vi "Write Future.vi"(8 "error in (no error)":errorcluster, 10 "Value":variant, 11 "Future in":refnum<class "Future.lvclass">) -> (0 "error out":errorcluster, 3 "Future out":refnum<class "Future.lvclass">)   [LabVIEW 2017, in "Promise Future.lvlib" / "Future.lvclass"]
uses:
  Future.lvclass
  Future.lvclass/Future.ctl
  c83e476c-f45e-459d-a1f3-ff7c88da77de.vi
  0608d02a-fc2f-4e6c-95dc-dd199133773d.vi
  Read Value.vi
  Value Set Callback.vi
  Wrapper VI Name.vi
  Then.vi
  <vilib>/Utility/error.llb/Error Cluster From Error Code.vi
  <vilib>/ErrorRing/Error Ring.xnode
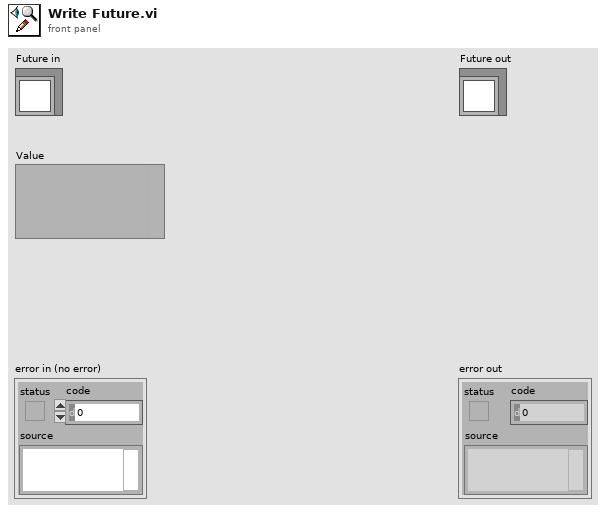
[diagram p1: front panel]
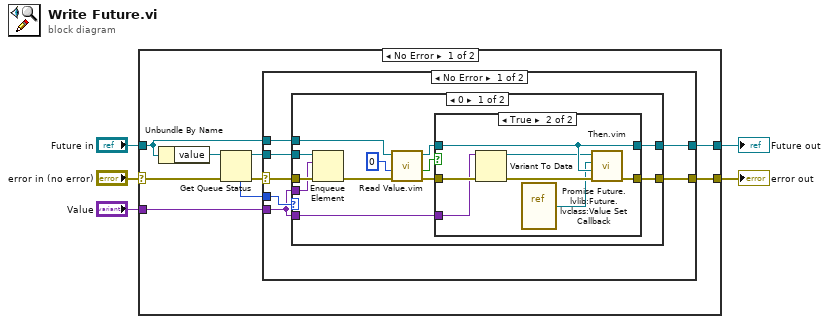
[diagram p0: block diagram]
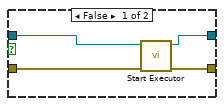
[diagram p2: hidden frame]
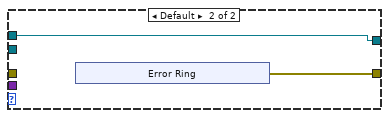
[diagram p3: hidden frame]
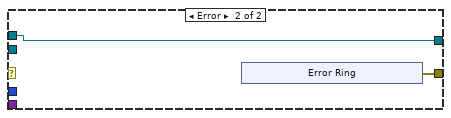
[diagram p4: hidden frame]
diagram:
  n1 = case shown="No Error" "error in (no error)" {
    selector: "error in (no error)" -> [w8 w60]
    tunnel: [w6 w60] -> w4
    tunnel: [w7 w59] -> w2
    tunnel: "Future in" -> [w10 w59]
    tunnel: "Value" -> [w9 _]
    frame No Error {
      n2 = Unbundle By Name(w10) -> ("value"=w11:refnum<queue>)
      n3 = Get Queue Status(queue=w11, error in (no error)=w8) -> (queue out=w13:refnum<queue>, error out=w14:errorcluster, # elements in queue=w12:i32)  [unwired: 1 in, 5 out]
      n4 = case shown="No Error" w14 {
        selector: w14 -> [w16 _]
        tunnel: [w21 w52] -> w6
        tunnel: w10 -> [w20 w53]
        tunnel: [w19 w53] -> w7
        tunnel: w12 -> [w18 _]
        tunnel: w13 -> [w17 _]
        tunnel: w9 -> [w15 _]
        frame No Error {
          n5 = case shown="0" w18 {
            tunnel: w20 -> [w28 w46]
            tunnel: w16 -> [w32 _]
            tunnel: [w29 w45] -> w21
            tunnel: [w30 w46] -> w19
            tunnel: w15 -> [w31 _]
            tunnel: w17 -> [w33 _]
            tunnel: w15 -> [w22 _]
            frame 0 {
              n6 = Enqueue Element(queue=w33, element=w31, error in (no error)=w32) -> (error out=w27:errorcluster)  [unwired: 1 in, 2 out]
              n7 = call "Read Value.vim"("error in (no error)"=w27, "timeout in ms (-1)"=0, "Future in"=w28) -> ("error out"=w26:errorcluster, "timed out?"=w24:bool, "Future out"=w25:refnum<class "Future.lvclass">)  [unwired: 5 in, 1 out]
              n8 = case shown="True" w24 {
                tunnel: [w37 w44] -> w30
                tunnel: [w36 w43] -> w29
                tunnel: w26 -> [w35 w41]
                tunnel: w25 -> [w34 w44]
                tunnel: w22 -> [_ w39]
                frame False {
                  n9 = call "Start Executor.vi"("error in (no error)"=w35, "Future in"=w34) -> ("error out"=w36:errorcluster, "Future out"=w37:refnum<class "Future.lvclass">)  [unwired: 8 in]
                }
                frame True {
                  n10 = Variant To Data(error in=w41, Variant=w39) -> (data=w40:refnum<class "Future.lvclass">, error out=w42:errorcluster)  [unwired: 1 in]
                  n11 = vi-ref "Promise Future.lvlib:Future.lvclass:Value Set Callback.vi"() -> (w38:refnum<vi>)
                  n12 = call "Then.vim"("error in (no error)"=w42, "Scope"=w44, "VI"=w38, "Future in"=w40) -> ("error out"=w43:errorcluster)  [unwired: 6 in, 1 out]
                }
              }
            }
            frame Default {
              n13 = xnode "Error Ring"() -> ("error out"=w45:errorcluster)
            }
          }
        }
        frame Error {
          n14 = xnode "Error Ring"() -> ("error out"=w52:errorcluster)
        }
      }
    }
    frame Error {
    }
  }
  "error out" <- w4
  "Future out" <- w2
